vi "Set Enable State on Multiple Controls.vi"(9 "Visible?":bool=TRUE, 10 "Enable?":bool=TRUE, 11 "Controls":refnum<vi>[](array[refnum])) -> ()   [LabVIEW 2015]
doc: "Sets all the controls in the input array to the \"Enable state\" value."
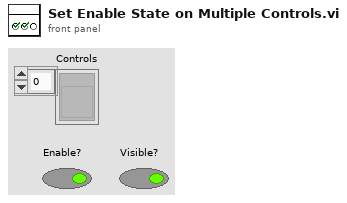
[diagram p1: front panel]
types:
  T1 = enum8{"Enabled", "Disabled", "Disabled and Grayed Out"}
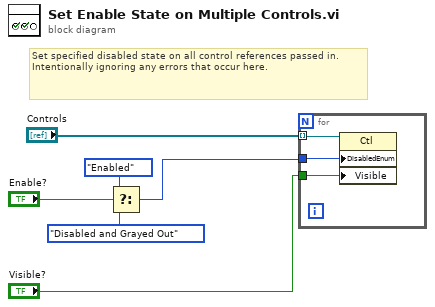
[diagram p0: block diagram]
diagram:
  # "Set specified disabled state on all control references passed in. Intentionally ignoring any errors that occur here."
  n1 = Select(t=T1."Enabled" ("Disabled"), s="Enable?", f=T1."Disabled and Grayed Out" ("Disabled")) -> (s? t:f=w4:T1)
  n2 = for {
    tunnel: "Controls" -> [w9] mode=indexing
    tunnel: w4 -> [w8]
    tunnel: "Visible?" -> [w7]
    n3 = property class="Ctl"(reference=w9, "DisabledEnum"=w8, "Visible"=w7) -> ()  [unwired: 1 in, 2 out]
  }
